vi "data_selection_and_analysis.vi"(8 "error in":errorcluster, 10 "days":i32, 11 "wind data in":dbl[][](array[numeric])) -> (0 "error out":errorcluster, 2 "sliding_panel_right":T1={"title"="Select a city", "Wind"=[]}, 3 "left_pane_cluster":T3={"title"="Select a city (# days)", "Power"=[], "max_power_slide"=0.0, "max_power_digi"=0.0, "max_power_title"="Select a city (# days)"} {"max_power_digi" format="%#_3g"; "max_power_slide" scale=0.0..40.0})   [LabVIEW 2020]
uses:
  controls/sliding_panel_left.ctl
  controls/power_chart.ctl
  controls/max_power_slider.ctl
  controls/sliding_panel_right.ctl
  controls/wind_chart.ctl
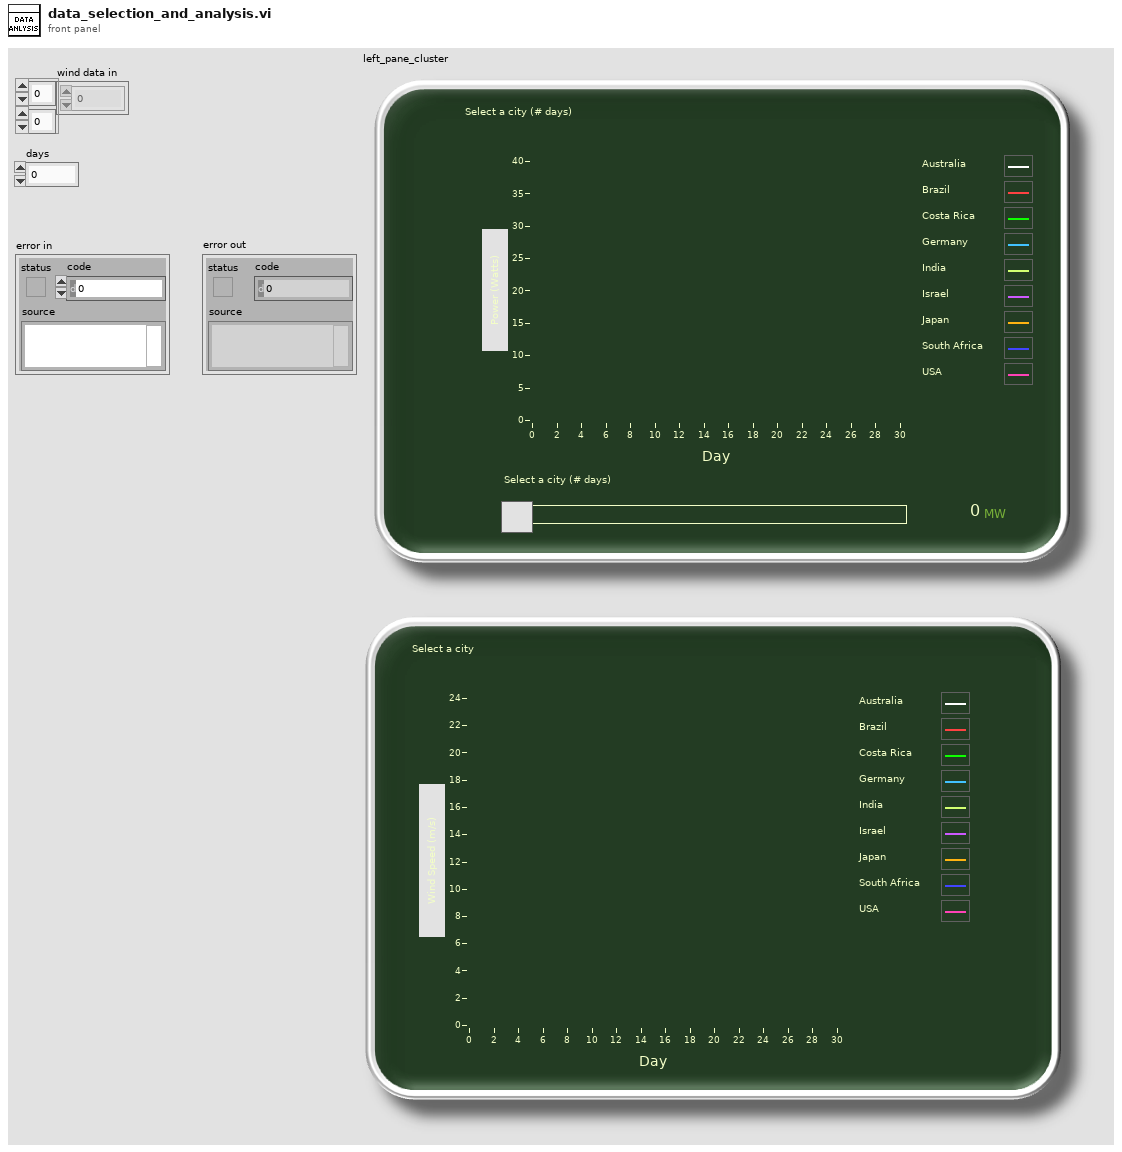
[diagram p1: front panel]
types:
  T1 = typedef "sliding_panel_right.ctl" = cluster{"title":string, "Wind":T2}
  T2 = typedef "wind_chart.ctl" = dbl[][]
  T3 = typedef "sliding_panel_left.ctl" = cluster{"title":string, "Power":T4, "max_power_slide":T5, "max_power_digi":dbl, "max_power_title":string}
  T4 = typedef "power_chart.ctl" = dbl[][]
  T5 = typedef "max_power_slider.ctl" = dbl
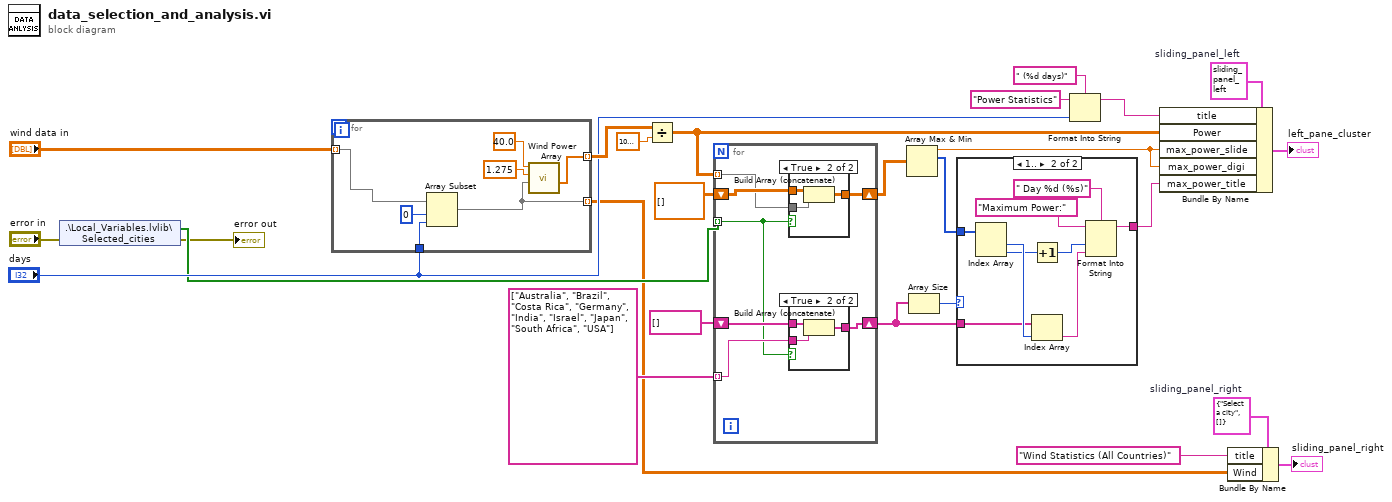
[diagram p0: block diagram]
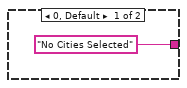
[diagram p2: hidden frame]
diagram:
  w6 = T1 {"title"="Select a city", "Wind"=[]}  # sliding_panel_right
  w22 = T3 {"title"="Power Statistics", "Power"=[], "max_power_slide"=3.1127450980392157, "max_power_digi"=130000.0, "max_power_title"=""}  # sliding_panel_left
  n1 = shared-variable ".\\Local_Variables.lvlib\\Selected_cities"(error in="error in") -> (w12:bool[], error out=→"error out":errorcluster)
  n2 = for {
    tunnel: "wind data in" -> [w27] mode=indexing
    tunnel: [w29] -> w3 mode=indexing
    tunnel: [w31] -> w24 mode=indexing
    tunnel: "days" -> [w28]
    n3 = Array Subset(array=w27, index=0, length=w28) -> (w29:dbl[])
    n4 = call "Wind Power Array.vi"("Wind Speed (m/s)"=w29, "Density (kg/m^3)"=1.275 ("Density"), "Blade Length (m)"=40.0 ("Blade Lenth")) -> ("Power (watts)"=w31:dbl[])  [unwired: 8 in]
  }
  n5 = Divide(x=w24, y=1000000.0 ("Blade Lenth")) -> (x/y=w13:dbl[][])
  n6 = for {
    tunnel: w13 -> [w38] mode=indexing
    shift-right: [w39] -> w11
    shift-left: dbl[][] [] -> [w40]
    tunnel: w12 -> [w34] mode=indexing
    tunnel: string[] ["Australia", "Brazil", "Costa Rica", "Germany", "India", "Israel", "Japan", "South Africa", "USA"] -> [w35] mode=indexing
    shift-right: [w37] -> w2
    shift-left: string[] [] -> [w36]
    n7 = case shown="True" w34 {
      tunnel: w38 -> [_ w48]
      tunnel: w40 -> [w45 w47]
      tunnel: [w45 w46] -> w39
      frame False {
      }
      frame True {
        n8 = Build Array (concatenate)(w47, w48) -> (w46:dbl[][])
      }
    }
    n9 = case shown="True" w34 {
      tunnel: w35 -> [_ w44]
      tunnel: w36 -> [w41 w43]
      tunnel: [w41 w42] -> w37
      frame False {
      }
      frame True {
        n10 = Build Array (concatenate)(w43, w44) -> (w42:string[])
      }
    }
  }
  n11 = Array Max & Min(array=w11) -> (max value=w21:dbl, max index (indices)=w15:i32[])  [unwired: 2 out]
  n12 = Array Size(array=w2) -> (size(s)=w1:i32)
  n13 = case shown="1.." w1 {
    tunnel: w15 -> [_ w56]
    tunnel: ["No Cities Selected" w55] -> w14
    tunnel: w2 -> [_ w52]
    frame 0, Default {
    }
    frame 1.. {
      n14 = Index Array(array=w56) -> (element #1=w54:i32, element #2=w53:i32)  [unwired: 2 in]
      n15 = Increment(x=w53) -> (x+1=w51:i32)
      n16 = Index Array(array=w52, index=w54) -> (element=w50:string)
      n17 = Format Into String(format string=" Day %d (%s)" ("initial string"), initial string="Maximum Power:", w51, w50) -> (resulting string=w55:string)  [unwired: 1 in, 1 out]
    }
  }
  n18 = Format Into String(format string=" (%d days)", initial string="Power Statistics", "days") -> (resulting string=w20:string)  [unwired: 1 in, 1 out]
  n19 = Bundle By Name(cluster=w22, "title"=w20, "Power"=w13, "max_power_slide"=w21, "max_power_digi"=w21, "max_power_title"=w14) -> (→"left_pane_cluster":T3)
  n20 = Bundle By Name(cluster=w6, "title"="Wind Statistics (All Countries)" ("initial string"), "Wind"=w3) -> (→"sliding_panel_right":T1)
